vi "LogDBIntegerChangeArray.vi"(4 "db connection":bool, 5 "names":string[](array[string]), 6 "current time":timestamp, 7 "prefix":string, 8 "error in (no error)":errorcluster, 9 "shift reg in":u32[](array[numeric]), 10 "values":u32[](array[numeric]), 11 "Refnum in":T1) -> (0 "error out":errorcluster, 1 "shift reg out":u32[](array[numeric]), 2 "db connection":bool, 3 "Refnum out":T1)   [LabVIEW 2011]
uses:
  <vilib>/addons/database/Connection.llb/Conn ObjectReference.ctl
  <vilib>/Utility/error.llb/DialogType.ctl
  <vilib>/addons/database/NI_Database_API.lvlib
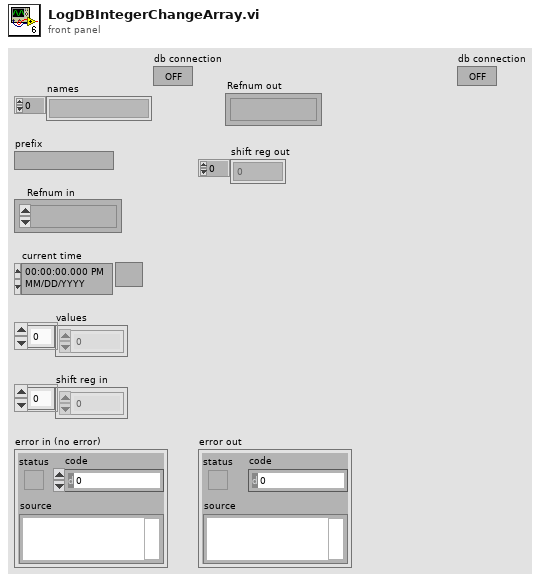
[diagram p1: front panel]
types:
  T1 = typedef "NI_Database_API.lvlib/Conn ObjectReference.ctl" = refnum<k1>
  T2 = typedef "DialogType.ctl" = u16
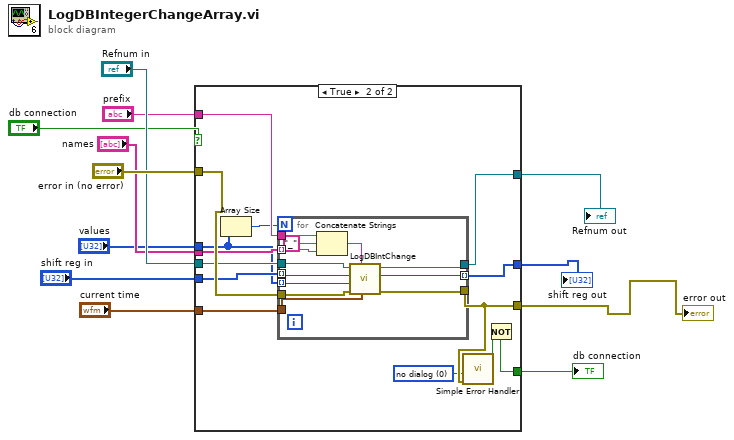
[diagram p0: block diagram]
diagram:
  n1 = case shown="True" "db connection" {
    selector: "db connection" -> [w13 _]
    tunnel: "current time" -> [_ w30]
    tunnel: "error in (no error)" -> [w14 w29]
    tunnel: "Refnum in" -> [w16 w28]
    tunnel: "prefix" -> [_ w27]
    tunnel: "names" -> [_ w26]
    tunnel: "shift reg in" -> [w15 w25]
    tunnel: "values" -> [_ w24]
    tunnel: [w15 w22] -> w5
    tunnel: [w16 w21] -> w4
    tunnel: [w14 w20] -> w2
    tunnel: [w13 w17] -> w1
    frame False {
    }
    frame True {
      w19 = T2 0 items=["no dialog", "OK message", "continue or stop message", "OK message + warnings", "continue/stop + warnings"] ("type of dialog (OK msg:1)")
      n2 = Array Size(array=w24) -> (size(s)=w23:i32)
      n3 = for {
        N: w23 -> [_]
        tunnel: [w40] -> w20
        tunnel: [w39] -> w21
        tunnel: [w38] -> w22 mode=indexing
        tunnel: w27 -> [w37]
        tunnel: w26 -> [w36] mode=indexing
        tunnel: w24 -> [w35] mode=indexing
        tunnel: w25 -> [w34] mode=indexing
        tunnel: w28 -> [w33]
        tunnel: w29 -> [w32]
        tunnel: w30 -> [w31]
        n4 = Concatenate Strings(w37, "_" ("string"), w36) -> (w41:string)
        n5 = call "LogDBIntChange.vi"("current time"=w31, "db table name"=w41, "error in"=w32, "value"=w35, "shiftReg"=w34, "Refnum in"=w33) -> ("error out"=w40:errorcluster, "shiftReg"=w38:u32, "Refnum out"=w39:T1)  [unwired: 3 in]
      }
      n6 = call <vilib>:"Simple Error Handler.vi"("type of dialog (OK msg:1)"=w19, "error in (no error)"=w20) -> ("error?"=w18:bool)  [unwired: 3 in, 4 out]
      n7 = Not(x=w18) -> (.not. x?=w17:bool)
    }
  }
  "error out" <- w2
  "Refnum out" <- w4
  "shift reg out" <- w5
  "db connection" <- w1
